vi "Plot Clip.vi"(7 "Clip Data":bool=TRUE, 8 "error in (no error)":errorcluster, 9 "Actual Transform In":T1, 11 "Plot Object In":refnum<vi>) -> (0 "error out":errorcluster, 1 "Actual Transform Out":T1, 3 "Plot Object Out":refnum<vi>)   [LabVIEW 2017, in "3D Plot.lvclass"]
uses:
  <vilib>/Math Plots/3D Math Plots/3D Plot/3D Plot/3D Plot.lvclass
  <vilib>/Math Plots/3D Math Plots/3D Plot/3D Plot/Typedef/Actual Transform.ctl
  <vilib>/Math Plots/3D Math Plots/3D Plot/3D Plot/Typedef/Range Clusters.ctl
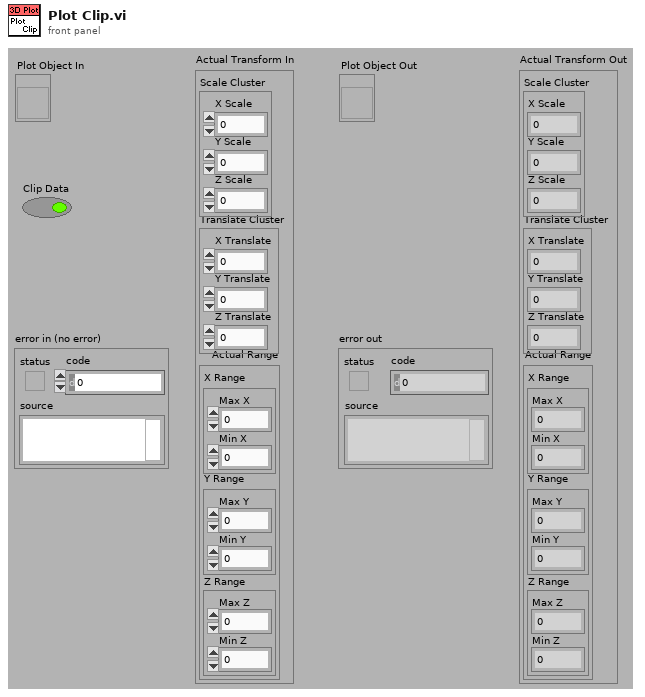
[diagram p1: front panel]
types:
  T1 = typedef "3D Plot.lvclass/Actual Transform.ctl" = cluster{"Scale Cluster":cluster{"X Scale":sgl, "Y Scale":sgl, "Z Scale":sgl}, "Translate Cluster":cluster{"X Translate":sgl, "Y Translate":sgl, "Z Translate":sgl}, "Actual Range":T2}
  T2 = typedef "3D Plot.lvclass/Range Clusters.ctl" = cluster{"X Range":cluster{"Max X":sgl, "Min X":sgl}, "Y Range":cluster{"Max Y":sgl, "Min Y":sgl}, "Z Range":cluster{"Max Z":sgl, "Min Z":sgl}}
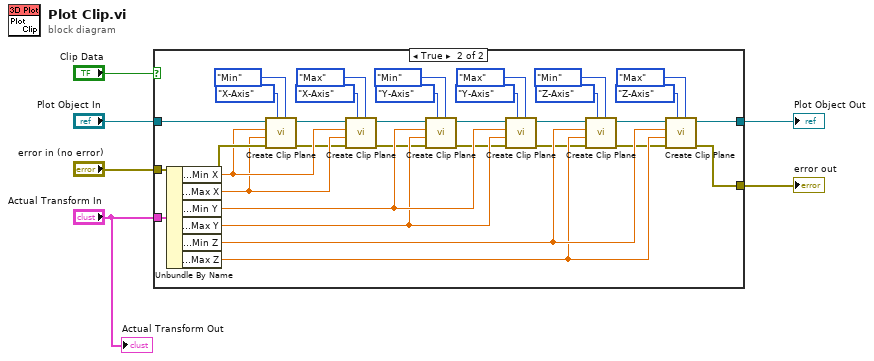
[diagram p0: block diagram]
diagram:
  n1 = case shown="True" "Clip Data" {
    tunnel: "Plot Object In" -> [w8 w40]
    tunnel: [w8 w15] -> w5
    tunnel: [w7 w9] -> w4
    tunnel: "Actual Transform In" -> [_ w41]
    tunnel: "error in (no error)" -> [w7 w39]
    frame False {
    }
    frame True {
      n2 = Unbundle By Name(w41) -> ("Actual Range.X Range.Min X"=w26:sgl, "Actual Range.X Range.Max X"=w25:sgl, "Actual Range.Y Range.Min Y"=w24:sgl, "Actual Range.Y Range.Max Y"=w23:sgl, "Actual Range.Z Range.Min Z"=w22:sgl, "Actual Range.Z Range.Max Z"=w21:sgl)
      n3 = call <vilib>:"Create Clip Plane.vi"("Type"=enum16{"Max", "Min"}."Min", "Axis"=enum16{"X-Axis", "Y-Axis", "Z-Axis"}."X-Axis", "error in (no error)"=w39, "Max"=w25, "Min"=w26, "Plot Object In"=w40) -> ("error out"=w14:errorcluster, "Plot Object Out"=w20:refnum<vi>)  [unwired: 4 out]
      n4 = call <vilib>:"Create Clip Plane.vi"("Type"=enum16{"Max", "Min"}."Max", "Axis"=enum16{"X-Axis", "Y-Axis", "Z-Axis"}."X-Axis", "error in (no error)"=w14, "Max"=w25, "Min"=w26, "Plot Object In"=w20) -> ("error out"=w13:errorcluster, "Plot Object Out"=w19:refnum<vi>)  [unwired: 4 out]
      n5 = call <vilib>:"Create Clip Plane.vi"("Type"=enum16{"Max", "Min"}."Min", "Axis"=enum16{"X-Axis", "Y-Axis", "Z-Axis"}."Y-Axis", "error in (no error)"=w13, "Max"=w23, "Min"=w24, "Plot Object In"=w19) -> ("error out"=w12:errorcluster, "Plot Object Out"=w18:refnum<vi>)  [unwired: 4 out]
      n6 = call <vilib>:"Create Clip Plane.vi"("Type"=enum16{"Max", "Min"}."Max", "Axis"=enum16{"X-Axis", "Y-Axis", "Z-Axis"}."Y-Axis", "error in (no error)"=w12, "Max"=w23, "Min"=w24, "Plot Object In"=w18) -> ("error out"=w11:errorcluster, "Plot Object Out"=w17:refnum<vi>)  [unwired: 4 out]
      n7 = call <vilib>:"Create Clip Plane.vi"("Type"=enum16{"Max", "Min"}."Min", "Axis"=enum16{"X-Axis", "Y-Axis", "Z-Axis"}."Z-Axis", "error in (no error)"=w11, "Max"=w21, "Min"=w22, "Plot Object In"=w17) -> ("error out"=w10:errorcluster, "Plot Object Out"=w16:refnum<vi>)  [unwired: 4 out]
      n8 = call <vilib>:"Create Clip Plane.vi"("Type"=enum16{"Max", "Min"}."Max", "Axis"=enum16{"X-Axis", "Y-Axis", "Z-Axis"}."Z-Axis", "error in (no error)"=w10, "Max"=w21, "Min"=w22, "Plot Object In"=w16) -> ("error out"=w9:errorcluster, "Plot Object Out"=w15:refnum<vi>)  [unwired: 4 out]
    }
  }
  "Plot Object Out" <- w5
  "error out" <- w4
  "Actual Transform Out" <- "Actual Transform In"
